vi "sub_psk_demod.vi"(8 "index map":i32[](array[numeric]), 9 "symbol map":cdb[](array[numeric]), 11 "symbol":cdb[](array[numeric])) -> (3 "bitstream":i16[](array[numeric]))   [LabVIEW 2014]
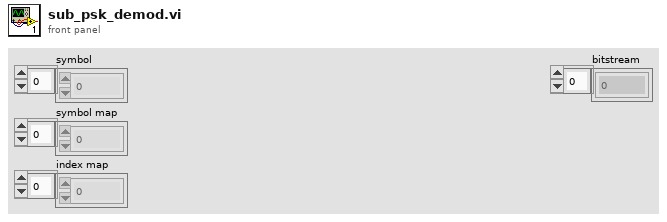
[diagram p1: front panel]
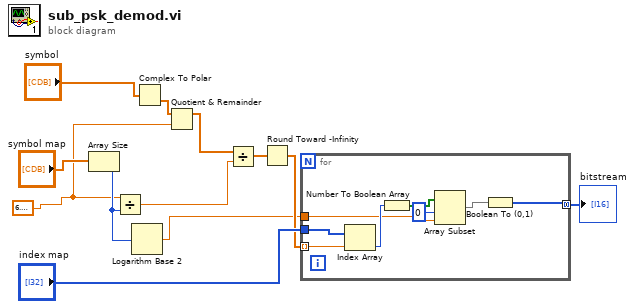
[diagram p0: block diagram]
diagram:
  w2 = 6.283185307179586
  n1 = Array Size(array="symbol map") -> (size(s)=w6:i32)
  n2 = Divide(x=w2, y=w6) -> (x/y=w10:dbl)
  n3 = Logarithm Base 2(1:w6) -> (0:w5:dbl)
  n4 = Complex To Polar(r * e^(i*theta)="symbol") -> (theta=w3:dbl[])  [unwired: 1 out]
  n5 = Quotient & Remainder(x=w3, y=w2) -> (x-y*floor(x/y)=w1:dbl[])  [unwired: 1 out]
  n6 = Divide(x=w1, y=w10) -> (x/y=w9:dbl[])
  n7 = Round Toward -Infinity(1:w9) -> (0:w7:dbl[])
  n8 = for {
    tunnel: "index map" -> [w20]
    tunnel: w7 -> [w19] mode=indexing
    tunnel: w5 -> [w16]
    tunnel: [w13] -> w4 mode=concatenating
    n9 = Index Array(array=w20, index=w19) -> (element=w18:i32)
    n10 = Number To Boolean Array(number=w18) -> (Boolean array=w17:bool[])
    n11 = Array Subset(array=w17, index=0, length=w16) -> (w14:bool[])
    n12 = Boolean To (0,1)(Boolean=w14) -> (0, 1=w13:i16[])
  }
  "bitstream" <- w4
